vi "ANAL_UpdateIndex.vi"(7 "ID Added":u32, 11 "GUI Cluster in":T1) -> (3 "GUI Cluster out":T1)   [LabVIEW 2021]
uses:
  ANAL_GUIStatus.ctl
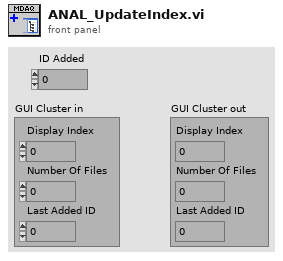
[diagram p1: front panel]
types:
  T1 = typedef "ANAL_GUIStatus.ctl" = cluster{"Display Index":i32, "Number Of Files":u32, "Last Added ID":u32}
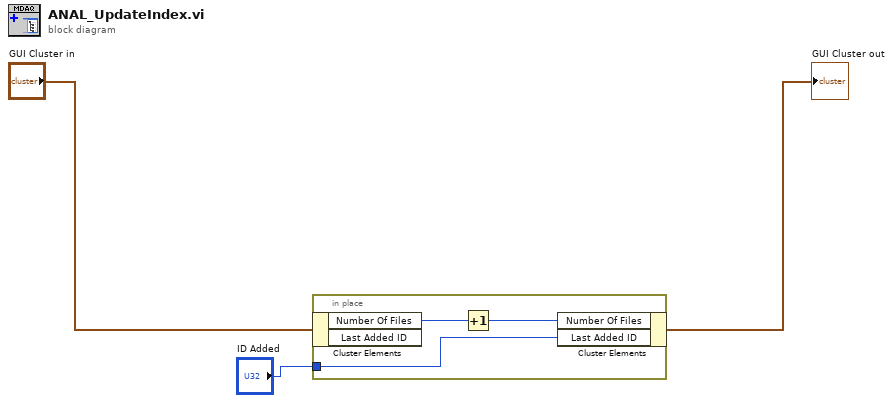
[diagram p0: block diagram]
diagram:
  n1 = in-place {
    in-place-border: "ID Added" -> [w4]
    n2 = in-place-cluster #1("GUI Cluster in") -> ("Number Of Files"=w6:u32)  [unwired: 1 out]
    n3 = Increment(x=w6) -> (x+1=w5:u32)
    n4 = in-place-cluster #1("Number Of Files"=w5, "Last Added ID"=w4) -> (→"GUI Cluster out":T1)
  }
